vi "Init.vi"(8 "error in (no error)":errorcluster, 10 "Error Log Path":path, 11 "Text Log in":refnum<class "Text Log.lvclass">) -> (0 "error out":errorcluster, 3 "Text Log out":refnum<class "Text Log.lvclass">)   [LabVIEW 2020, in "Error Log Classes.lvlib" / "Text Log.lvclass"]
uses:
  Text Log.lvclass
  Text Log.lvclass/Text Log.ctl
  Error Log/Error Log.lvclass
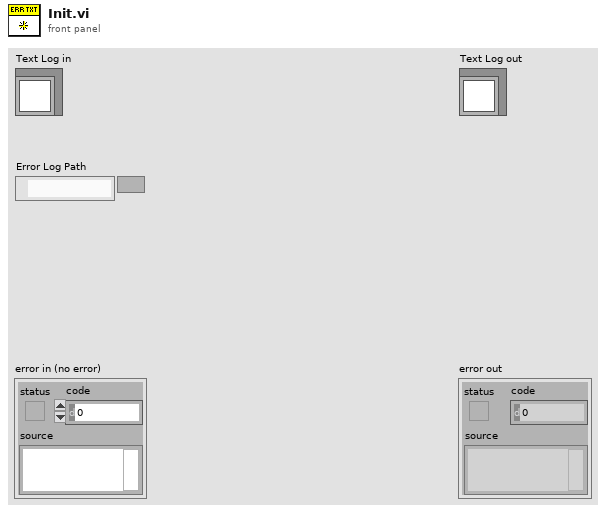
[diagram p1: front panel]
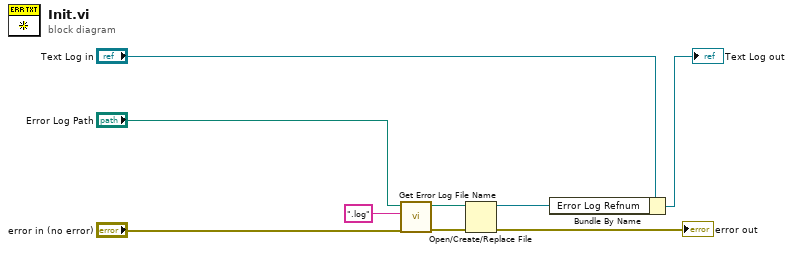
[diagram p0: block diagram]
diagram:
  n1 = call "Get Error Log File Name.vi"("error in (no error)"="error in (no error)", "Extension"=".log" ("string"), "Error Log Path in"="Error Log Path") -> ("error out"=w6:errorcluster, "Error Log Path out"=w8:path)  [unwired: 7 in]
  n2 = Open/Create/Replace File(file path (use dialog)=w8, error in=w6) -> (refnum out=w2:refnum<file>, error out=→"error out":errorcluster)  [unwired: 4 in, 1 out]
  n3 = Bundle By Name(cluster="Text Log in", "Error Log Refnum"=w2) -> (→"Text Log out":refnum<class "Text Log.lvclass">)
